vi "pitcher.vi"() -> ()   [LabVIEW 2012, in "Matura.lvrbt"]
uses:
  Desktop/Matura/Matura.lvrbt
  <vilib>/NXT/NXT Controls/ConnectionType.ctl
panel:
  in  "stop":bool
  in  "Tonhšhe 2":u16=440
  in  "Tonhšhe 1":u16=440
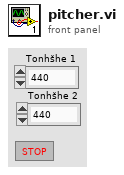
[diagram p1: front panel]
types:
  T1 = typedef "ConnectionType.ctl" = enum16{"Bluetooth", "USB", "WiFi"}
  T2 = typedef "LVHSConnector.ctl" = refnum<class "BrickReference.lvclass">
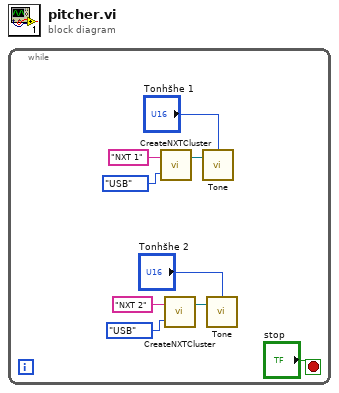
[diagram p0: block diagram]
diagram:
  n1 = while {
    stop <- "stop" stop-if-true
    n2 = call <vilib>:"CreateNXTCluster.vi"("Connection Type"=ConnectionType."USB", "NXT name"="NXT 1") -> ("NXT"=w4:T2)  [unwired: 2 in]
    n3 = call <vilib>:"CreateNXTCluster.vi"("Connection Type"=ConnectionType."USB", "NXT name"="NXT 2") -> ("NXT"=w5:T2)  [unwired: 2 in]
    n4 = call <vilib>:"Tone.vi"("NXT"=w4, "Tone (440 Hz)"="Tonhšhe 1") -> ()  [unwired: 2 in, 1 out]
    n5 = call <vilib>:"Tone.vi"("NXT"=w5, "Tone (440 Hz)"="Tonhšhe 2") -> ()  [unwired: 2 in, 1 out]
  }
